vi "Category Manager.vi"(8 "error in (no error)":errorcluster, 11 "Budgetizer.lvclass":refnum<class "Budgetizer.lvclass">) -> (0 "error out":errorcluster, 3 "Budgetizer.lvclass":refnum<class "Budgetizer.lvclass">)   [LabVIEW 2018]
uses:
  support/classes/Budgetizer/Budgetizer.lvclass
  support/classes/Category/Category.lvclass
panel:
  in  "Rename":bool
  in  "Delete":bool
  in  "Close":bool
  in  "Add":bool
  in  "Category Name":string
  in  "Category Table":i32(listbox)
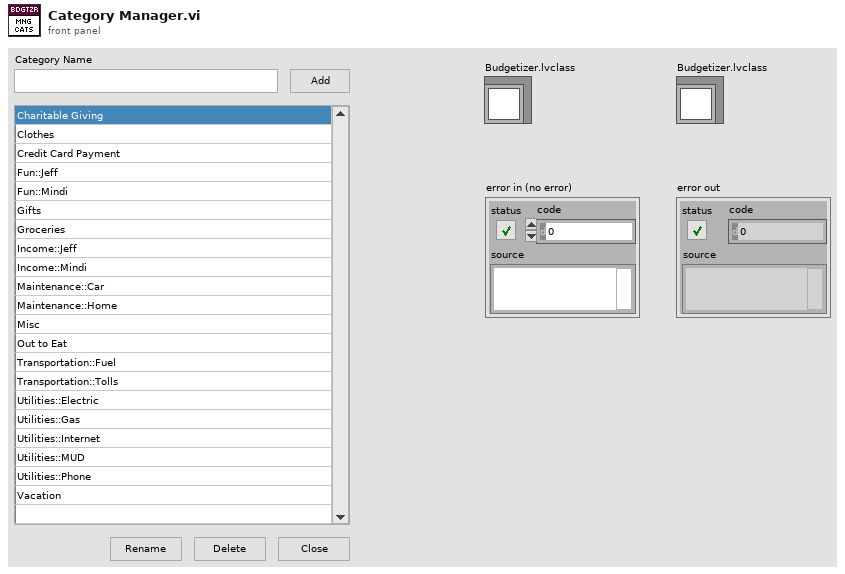
[diagram p1: front panel]
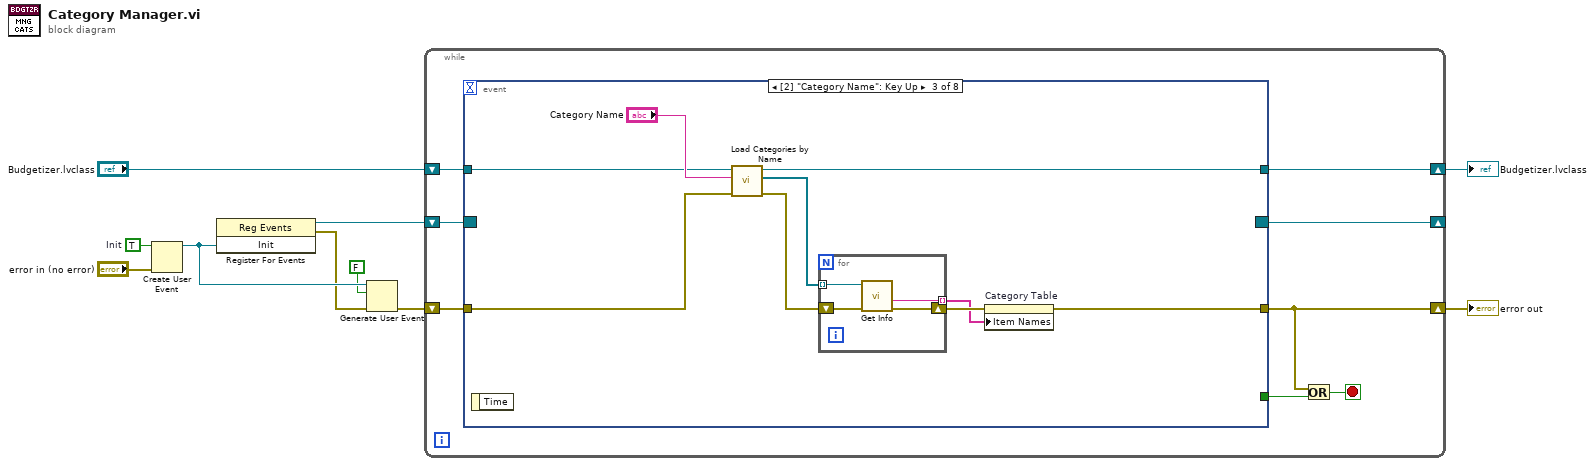
[diagram p0: block diagram]
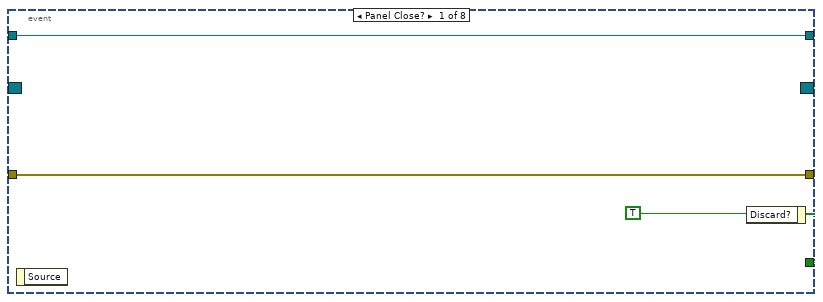
[diagram p2: hidden frame]
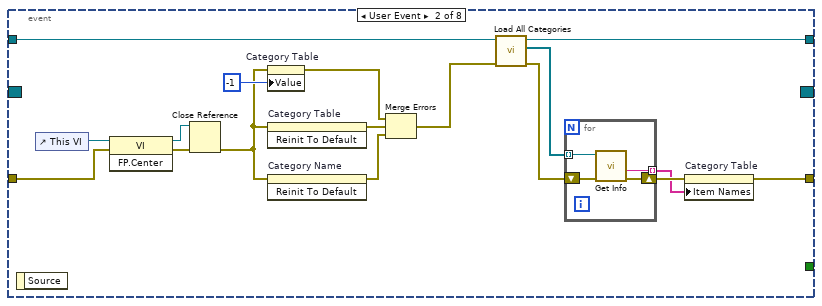
[diagram p3: hidden frame]
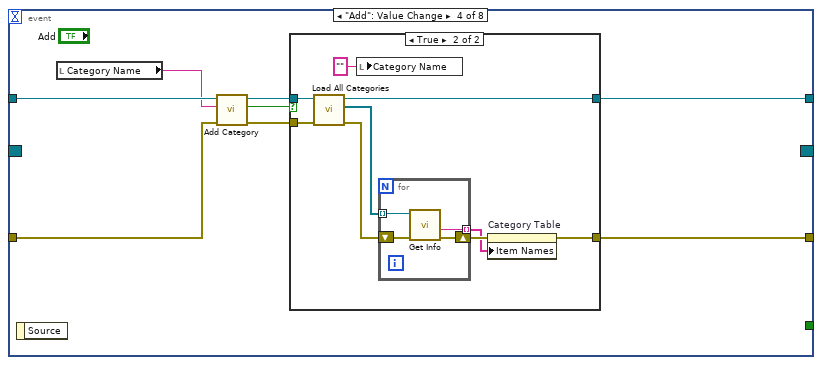
[diagram p4: hidden frame]
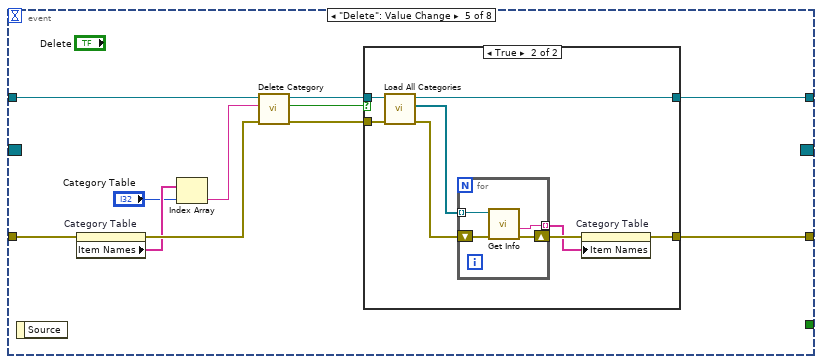
[diagram p6: hidden frame]
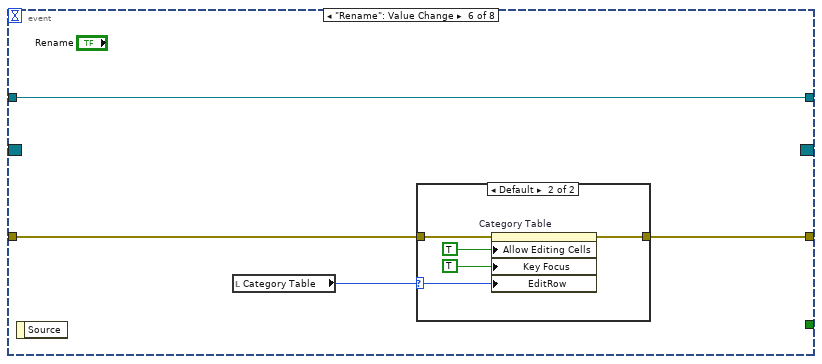
[diagram p8: hidden frame]
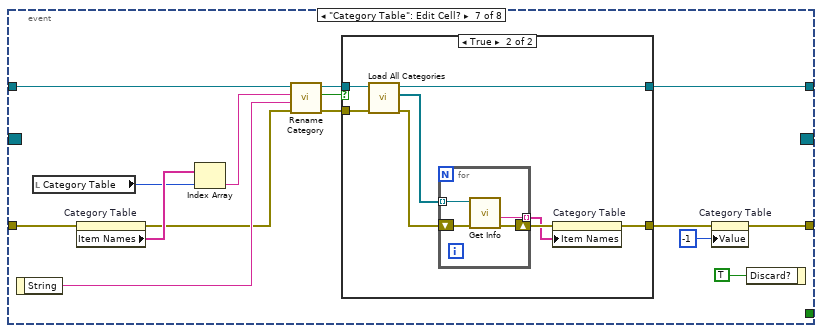
[diagram p10: hidden frame]
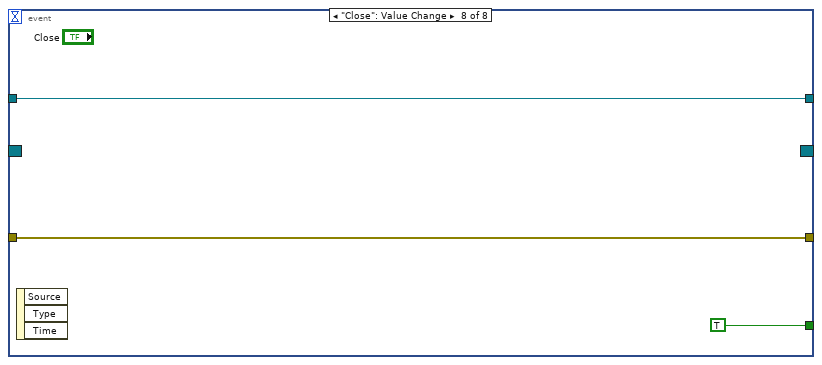
[diagram p12: hidden frame]
diagram:
  w10 = TRUE  # Init
  n1 = Create User Event(user event datatype=w10, error in="error in (no error)") -> (user event=w8:refnum<user-event>)  [unwired: 1 out]
  n2 = register-events(w8) -> (reference out=w9:refnum<event-registration>, error out=w7:errorcluster)  [unwired: 2 in]
  n3 = Generate User Event(user event=w8, event data cluster=FALSE ("event data"), error in=w7) -> (error out=w6:errorcluster)  [unwired: 1 in, 1 out]
  n4 = while {
    shift-right: [w16] -> _
    shift-left: w9 -> [w18]
    shift-right: [w13] -> w1
    shift-left: w6 -> [w17]
    shift-right: [w14] -> w2
    shift-left: "Budgetizer.lvclass" -> [w15]
    stop <- w11 stop-if-true
    n5 = event shown="[2] \"Category Name\": Key Up" {
      selector: w18 -> [_ _ _ _ _ _ _ _]
      dyn-events: [_ _ _ _ _ _ _ _] -> w16
      timeout: _ -> [_ _ _ _ _ _ _ _]
      tunnel: [w21 _ _ _ _ _ _ TRUE ("Discard?")] -> w12
      tunnel: w17 -> [w20 w33 w51 w62 w88 w107 w126 w145]
      tunnel: [w20 w36 w49 w57 w82 w106 w114 w145] -> w13
      tunnel: w15 -> [w19 w28 w48 w63 w89 w105 w125 w144]
      tunnel: [w19 w27 w47 w58 w80 w105 w117 w144] -> w14
      event Panel Close? {
        w21 = TRUE ("Discard?")
        n6 = event-data() -> ()  [unwired: 1 in, 1 out]
        n7 = event-data("Discard?"=w21) -> ()  [unwired: 1 in, 1 out]
      }
      event User Event {
        n8 = event-data() -> ()  [unwired: 1 in, 1 out]
        n9 = control-ref of="This VI"() -> (w34:refnum<vi>)
        n10 = invoke class="VI" method="FP.Center"(reference=w34, error in=w33) -> (reference out=w31:refnum<vi>, error out=w32:errorcluster)  [unwired: 1 in, 1 out]
        n11 = Close Reference(reference=w31, error in (no error)=w32) -> (error out=w30:errorcluster)
        n12 = property on="Category Table" class="LstBox (strict)"(error in=w30, "Value"=-1 ("Category Table")) -> (error out=w29:errorcluster)  [unwired: 1 in, 1 out]
        n13 = invoke on="Category Table" class="LstBox (strict)" method="Reinit To Default"(error in=w30) -> (error out=w37:errorcluster)  [unwired: 2 in, 2 out]
        n14 = invoke on="Category Name" class="Str" method="Reinit To Default"(error in=w30) -> (error out=w38:errorcluster)  [unwired: 2 in, 2 out]
        n15 = Merge Errors(w29, w37, w38) -> (w26:errorcluster)
        n16 = call "Load All Categories.vi"("error in (no error)"=w26, "Budgetizer in"=w28) -> ("error out"=w24:errorcluster, "Categories"=w23:refnum<class "Category.lvclass">[], "Budgetizer out"=w27:refnum<class "Budgetizer.lvclass">)  [unwired: 7 in]
        n17 = for {
          shift-right: [w42] -> w25
          shift-left: w24 -> [w41]
          tunnel: w23 -> [w40] mode=indexing
          tunnel: [w39] -> w22 mode=indexing
          n18 = call "Get Info.vi"("error in (no error)"=w41, "Category in"=w40) -> ("error out"=w42:errorcluster, "Name"=w39:string)  [unwired: 6 in, 2 out]
        }
        n19 = property on="Category Table" class="LstBox (strict)"(error in=w25, "Item Names"=w22) -> (error out=w36:errorcluster)  [unwired: 1 in, 1 out]
      }
      event "Category Name": Key Up {
        n20 = event-data() -> ()  [unwired: 1 in, 1 out]
        n21 = call "Load Categories by Name.vi"("error in (no error)"=w51, "String Input"="Category Name", "Budgetizer.lvclass"=w48) -> ("error out"=w45:errorcluster, "Matching Categories"=w46:refnum<class "Category.lvclass">[], "Budgetizer.lvclass"=w47:refnum<class "Budgetizer.lvclass">)  [unwired: 6 in]
        n22 = for {
          tunnel: w46 -> [w54] mode=indexing
          shift-right: [w53] -> w44
          shift-left: w45 -> [w55]
          tunnel: [w52] -> w43 mode=indexing
          n23 = call "Get Info.vi"("error in (no error)"=w55, "Category in"=w54) -> ("error out"=w53:errorcluster, "Name"=w52:string)  [unwired: 6 in, 2 out]
        }
        n24 = property on="Category Table" class="LstBox (strict)"(error in=w44, "Item Names"=w43) -> (error out=w49:errorcluster)  [unwired: 1 in, 1 out]
      }
      event "Add": Value Change {
        n25 = event-data() -> ()  [unwired: 1 in, 1 out]
        n26 = local read "Category Name"() -> (w61:string)
        n27 = call "Add Category.vi"("error in (no error)"=w62, "Category Name"=w61, "Budgetizer in"=w63) -> ("error out"=w59:errorcluster, "Anything Added?"=w56:bool, "Budgetizer out"=w60:refnum<class "Budgetizer.lvclass">)  [unwired: 6 in]
        n28 = case shown="True" w56 {
          tunnel: w60 -> [w65 w74]
          tunnel: w59 -> [w64 w73]
          tunnel: [w65 w71] -> w58
          tunnel: [w64 w72] -> w57
          frame False {
          }
          frame True {
            n29 = call "Load All Categories.vi"("error in (no error)"=w73, "Budgetizer in"=w74) -> ("error out"=w68:errorcluster, "Categories"=w67:refnum<class "Category.lvclass">[], "Budgetizer out"=w71:refnum<class "Budgetizer.lvclass">)  [unwired: 7 in]
            n30 = local write "Category Name"("" ("Category Name")) -> ()
            n31 = for {
              shift-right: [w78] -> w69
              shift-left: w68 -> [w77]
              tunnel: w67 -> [w76] mode=indexing
              tunnel: [w75] -> w66 mode=indexing
              n32 = call "Get Info.vi"("error in (no error)"=w77, "Category in"=w76) -> ("error out"=w78:errorcluster, "Name"=w75:string)  [unwired: 6 in, 2 out]
            }
            n33 = property on="Category Table" class="LstBox (strict)"(error in=w69, "Item Names"=w66) -> (error out=w72:errorcluster)  [unwired: 1 in, 1 out]
          }
        }
      }
      event "Delete": Value Change {
        n34 = event-data() -> ()  [unwired: 1 in, 1 out]
        n35 = property on="Category Table" class="LstBox (strict)"(error in=w88) -> (error out=w87:errorcluster, "Item Names"=w86:string[])  [unwired: 1 in, 1 out]
        n36 = Index Array(array=w86, index="Category Table") -> (element=w84:string)
        n37 = call "Delete Category.vi"("error in (no error)"=w87, "Category Name"=w84, "Budgetizer in"=w89) -> ("error out"=w83:errorcluster, "Anything Deleted?"=w79:bool, "Budgetizer out"=w81:refnum<class "Budgetizer.lvclass">)  [unwired: 6 in]
        n38 = case shown="True" w79 {
          tunnel: w81 -> [w91 w99]
          tunnel: w83 -> [w90 w98]
          tunnel: [w91 w96] -> w80
          tunnel: [w90 w97] -> w82
          frame False {
          }
          frame True {
            n39 = call "Load All Categories.vi"("error in (no error)"=w98, "Budgetizer in"=w99) -> ("error out"=w94:errorcluster, "Categories"=w93:refnum<class "Category.lvclass">[], "Budgetizer out"=w96:refnum<class "Budgetizer.lvclass">)  [unwired: 7 in]
            n40 = for {
              shift-right: [w103] -> w95
              shift-left: w94 -> [w102]
              tunnel: w93 -> [w101] mode=indexing
              tunnel: [w100] -> w92 mode=indexing
              n41 = call "Get Info.vi"("error in (no error)"=w102, "Category in"=w101) -> ("error out"=w103:errorcluster, "Name"=w100:string)  [unwired: 6 in, 2 out]
            }
            n42 = property on="Category Table" class="LstBox (strict)"(error in=w95, "Item Names"=w92) -> (error out=w97:errorcluster)  [unwired: 1 in, 1 out]
          }
        }
      }
      event "Rename": Value Change {
        n43 = event-data() -> ()  [unwired: 1 in, 1 out]
        n44 = local read "Category Table"() -> (w104:i32)
        n45 = case shown="Default" w104 {
          selector: w104 -> [_ w109]
          tunnel: w107 -> [w108 w113]
          tunnel: [w108 w111] -> w106
          frame ..-1 {
          }
          frame Default {
            n46 = property on="Category Table" class="LstBox (strict)"(error in=w113, "Allow Editing Cells"=TRUE, "Key Focus"=TRUE, "EditRow"=w109) -> (error out=w111:errorcluster)  [unwired: 1 in, 1 out]
          }
        }
      }
      event "Category Table": Edit Cell? {
        n47 = event-data() -> ("String"=w124:string)  [unwired: 1 in]
        n48 = local read "Category Table"() -> (w127:i32)
        n49 = property on="Category Table" class="LstBox (strict)"(error in=w126) -> (error out=w122:errorcluster, "Item Names"=w128:string[])  [unwired: 1 in, 1 out]
        n50 = Index Array(array=w128, index=w127) -> (element=w123:string)
        n51 = call "Rename Category.vi"("error in (no error)"=w122, "New Name"=w124, "Old Name"=w123, "Budgetizer in"=w125) -> ("error out"=w118:errorcluster, "Anything Renamed?"=w119:bool, "Budgetizer out"=w120:refnum<class "Budgetizer.lvclass">)  [unwired: 5 in]
        n52 = case shown="True" w119 {
          tunnel: w120 -> [w130 w138]
          tunnel: w118 -> [w129 w137]
          tunnel: [w130 w136] -> w117
          tunnel: [w129 w135] -> w115
          frame False {
          }
          frame True {
            n53 = call "Load All Categories.vi"("error in (no error)"=w137, "Budgetizer in"=w138) -> ("error out"=w133:errorcluster, "Categories"=w132:refnum<class "Category.lvclass">[], "Budgetizer out"=w136:refnum<class "Budgetizer.lvclass">)  [unwired: 7 in]
            n54 = for {
              shift-right: [w142] -> w134
              shift-left: w133 -> [w141]
              tunnel: w132 -> [w140] mode=indexing
              tunnel: [w139] -> w131 mode=indexing
              n55 = call "Get Info.vi"("error in (no error)"=w141, "Category in"=w140) -> ("error out"=w142:errorcluster, "Name"=w139:string)  [unwired: 6 in, 2 out]
            }
            n56 = property on="Category Table" class="LstBox (strict)"(error in=w134, "Item Names"=w131) -> (error out=w135:errorcluster)  [unwired: 1 in, 1 out]
          }
        }
        n57 = property on="Category Table" class="LstBox (strict)"(error in=w115, "Value"=-1 ("Category Table")) -> (error out=w114:errorcluster)  [unwired: 1 in, 1 out]
        n58 = event-data("Discard?"=TRUE) -> ()  [unwired: 1 in, 1 out]
      }
      event "Close": Value Change {
        n59 = event-data() -> ()  [unwired: 1 in, 3 out]
      }
    }
    n60 = Or(x=w13, y=w12) -> (x .or. y?=w11:bool)
  }
  "Budgetizer.lvclass" <- w2
  "error out" <- w1
